vi "L_Risize.vi"(2 "error in (no error)":errorcluster caption="错误输入（无错误）", 3 "本VI":refnum<vi>) -> (0 "error out":errorcluster caption="错误输出")   [LabVIEW 2012]
uses:
  <vilib>/Utility/inputDevices.llb/mouseAcquire.vi
  <vilib>/Utility/inputDevices.llb/closeMouse.vi
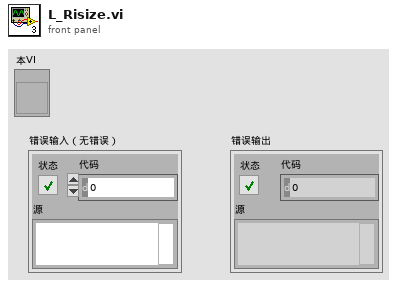
[diagram p1: front panel]
types:
  T1 = cluster{"Horizontal":i32, "Vertical":i32, "Scrolling":i32}
  T2 = cluster{"button 1":bool, "button 2":bool, "button 3":bool, "button 4":bool}
  T3 = typedef "LVRectTypeDef.ctl" = cluster{"Left":i16, "Top":i16, "Right":i16, "Bottom":i16}
  T4 = cluster{"Horizontal":i32, "Top":i16, "Right":i16, "Bottom":i16}
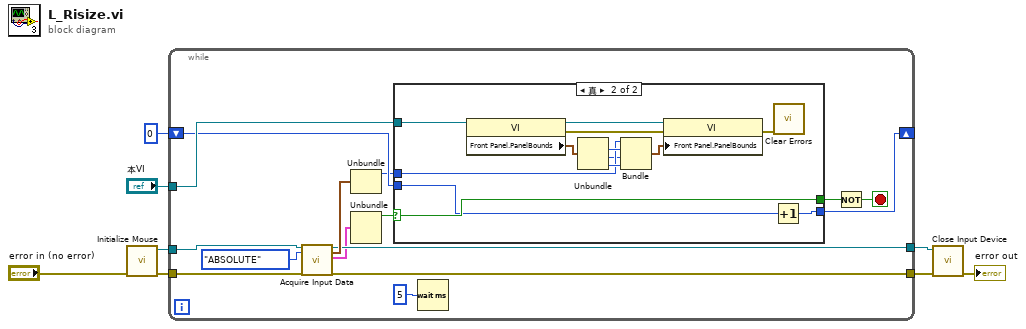
[diagram p0: block diagram]
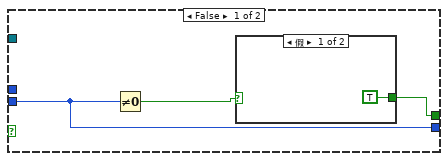
[diagram p2: hidden frame]
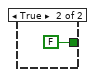
[diagram p3: hidden frame]
diagram:
  n1 = call <vilib>:"Initialize Mouse.vi"("error in (no error)"="error in (no error)") -> ("error out"=w7:errorcluster, "device ID"=w8:refnum<k1>)  [unwired: 9 in]
  n2 = while {
    tunnel: w8 -> [w22]
    tunnel: w7 -> [w21]
    tunnel: [w19] -> w6
    tunnel: [w18] -> w5
    tunnel: "本VI" -> [w14]
    shift-right: [w10] -> _
    shift-left: u32 0 ("等待时间（毫秒）") -> [w11]
    stop <- w12 stop-if-true
    n3 = call-poly <vilib>:"Acquire Input Data.vi"("device ID"=w22, "key mode"=enum16{"RELATIVE", "ABSOLUTE"}."ABSOLUTE", "error in (no error)"=w21) -> ("device ID"=w19:refnum<k1>, "axis info"=w20:T1, "button info"=w17:T2, "error out"=w18:errorcluster)  [unwired: 13 in]
    n4 = Unbundle(w20) -> ("Horizontal"=w9:i32)  [unwired: 2 out]
    n5 = Unbundle(w17) -> ("button 1"=w16:bool)  [unwired: 3 out]
    n6 = case shown="真" w16 {
      selector: w16 -> [_ w37]
      tunnel: w9 -> [_ w31]
      tunnel: w14 -> [_ w38]
      tunnel: [w26 w37] -> w13
      tunnel: w11 -> [w24 w36]
      tunnel: [w24 w35] -> w10
      frame False {
        n7 = Not Equal To 0?(x=w24) -> (x != 0?=w25:bool)
        n8 = case shown="假" w25 {
          tunnel: [TRUE FALSE] -> w26
          frame False {
          }
          frame True {
          }
        }
      }
      frame True {
        n9 = property class="VI"(reference=w38) -> (reference out=w41:refnum<vi>, error out=w34:errorcluster, "Front Panel.PanelBounds"=w40:T3)  [unwired: 1 in]
        n10 = Unbundle(w40) -> ("Top"=w32:i16, "Right"=w30:i16, "Bottom"=w33:i16)  [unwired: 1 out]
        n11 = Bundle("Horizontal"=w31, "Top"=w32, "Right"=w30, "Bottom"=w33) -> (w39:T4)  [unwired: 1 in]
        n12 = property class="VI"(reference=w41, error in=w34, "Front Panel.PanelBounds"=w39) -> (error out=w29:errorcluster)  [unwired: 1 out]
        n13 = Increment(x=w36) -> (x+1=w35:u32)
        n14 = call <vilib>:"Clear Errors.vi"("error in (no error)"=w29) -> ()  [unwired: 6 in, 1 out]
      }
    }
    n15 = Wait (ms)(milliseconds to wait=u32 5 ("等待时间（毫秒）")) -> ()  [unwired: 1 out]
    n16 = Not(x=w13) -> (.not. x?=w12:bool)
  }
  n17 = call-poly <vilib>:"Close Input Device.vi"("error in (no error)"=w5, "device ID"=w6) -> ("error out"=→"error out":errorcluster)  [unwired: 8 in]
